vi "Demo.vi"() -> ()   [LabVIEW 2014]
uses:
  Linked List/node/node.lvclass
panel:
  out "Array":dbl[](array[numeric])
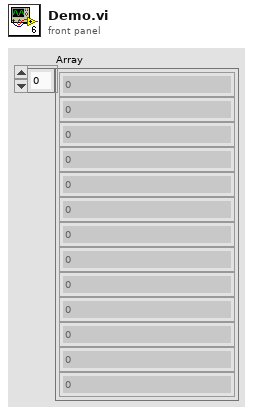
[diagram p1: front panel]
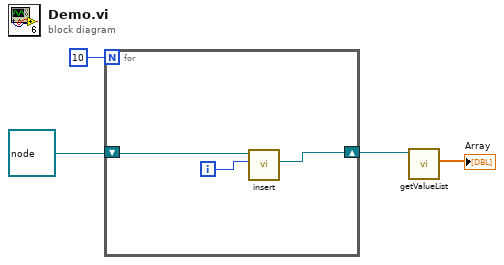
[diagram p0: block diagram]
diagram:
  n1 = for {
    N: 10 -> [_]
    shift-right: [w5] -> w3
    shift-left: refnum<class "node.lvclass"> refnum ("Linked List.lvlib:node") -> [w7]
    i -> [w6]
    n2 = call-dynamic "insert.vi"("data"=w6, "node in"=w7) -> ("pre"=w5:refnum<class "node.lvclass">)  [unwired: 7 in, 2 out]
  }
  n3 = call-dynamic "getValueList.vi"("node in"=w3) -> ("Array"=→"Array":dbl[])  [unwired: 8 in, 2 out]
